vi "Measure.vi"(8 "error in (no error)":errorcluster, 11 "B&K Precision 9120 series in":refnum<class "B&K Precision 9120 series.lvclass">) -> (0 "error out":errorcluster, 1 "Current":dbl, 2 "Voltage":dbl, 3 "B&K Precision 9120 series out":refnum<class "B&K Precision 9120 series.lvclass">)   [LabVIEW 2014, in "B&K Precision 9120 series.lvclass"]
uses:
  B&K Precision 9120 series.lvclass
  B&K Precision 9120 series.lvclass/B&K Precision 9120 series.ctl
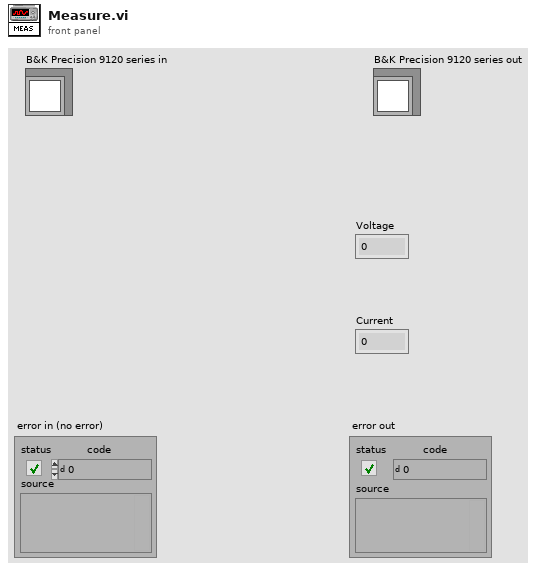
[diagram p1: front panel]
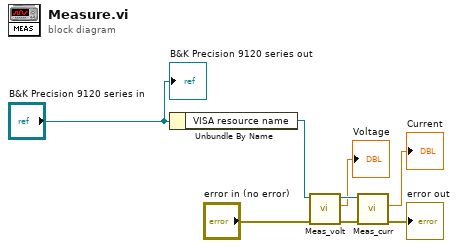
[diagram p0: block diagram]
diagram:
  n1 = Unbundle By Name("B&K Precision 9120 series in") -> ("VISA resource name"=w4:refnum<visa-resource-name>)
  n2 = call "Meas_volt.vi"("error in (no error)"="error in (no error)", "VISA resource in"=w4) -> ("error out"=w7:errorcluster, "Voltage"=→"Voltage":dbl, "VISA resource out"=w3:refnum<visa-resource-name>)  [unwired: 7 in]
  n3 = call "Meas_curr.vi"("error in (no error)"=w7, "VISA resource in"=w3) -> ("error out"=→"error out":errorcluster, "Current"=→"Current":dbl)  [unwired: 7 in, 1 out]
  "B&K Precision 9120 series out" <- "B&K Precision 9120 series in"
